vi "NIMS_DF_iir_grpdelay.vi"(5 "r":dbl=0.9999, 6 "w":dbl[](array[numeric]), 7 "grp":dbl[](array[numeric]), 9 "e":dbl[](array[numeric]), 10 "f":dbl[](array[numeric]), 11 "n":i32) -> (0 "error":i32, 1 "offset":dbl=0.9999, 2 "a":dbl[](array[numeric]), 3 "b":dbl[](array[numeric]))   [LabVIEW 2017, in "NI_DigFilter_MathScript.lvlib"]
uses:
  <vilib>/addons/Digital Filter Design/NI_DigFilter_MathScript.lvlib
  <vilib>/addons/Digital Filter Design/NI_DigFilterLicensed.lvlib
panel:
  in  "reserved4":dbl=nan
  in  "reserved3":dbl[](array[numeric])
  in  "reserved2":dbl=20.0
  in  "reserved1":i32[](array[numeric])=[2, 128]
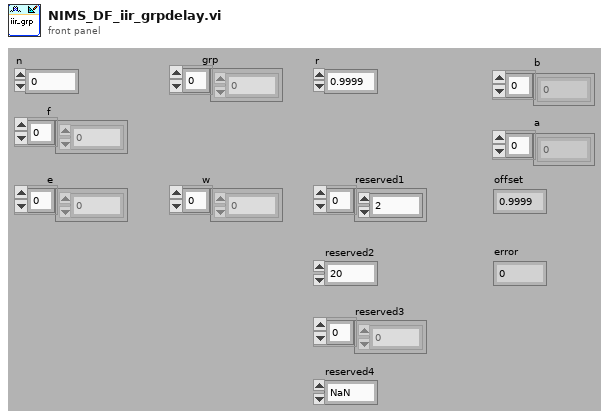
[diagram p1: front panel]
types:
  T1 = typedef "NI_DigFilterLicensed.lvlib/dfd_Group Delay_Band Spec.ctl" = cluster{"subband specs":cluster{"freq":dbl, "group delay":dbl, "weight":dbl}[]}
  T2 = typedef "NI_DigFilterLicensed.lvlib/DFD Filter Obj.ctl" = cluster{"mSRate_Fs":dbl, "mSRate_Version":string, "mSRate_Comments":string, "mSRate_OrgCoef":T3, "mSRate_CurCoef":T3, "mSRate_Quantized?":bool, "mSRate_QCoef":T3, "mSRate_QSettings":T5[], "mSRate_Order":i32, "mSRate_Scaling":cluster{"mSRate_ScaleByPowerOf2?":bool, "mSRate_ScaleType":T7}}
  T3 = typedef "NI_DigFilterLicensed.lvlib/DFD Filter Coef.ctl" = cluster{"type":T4, "gain":dbl, "coef a (k)":dbl[], "coef b (v)":dbl[]}
  T4 = typedef "NI_DigFilterLicensed.lvlib/DFD Filter Structure Type Selector.ctl" = enum16{"Undefined", "FIR Direct Form", "FIR Direct Form Transposed", "FIR Symmetric", "FIR Antisymmetric", "IIR Direct Form I", "IIR Direct Form I Transposed", "IIR Direct Form II", "IIR Direct Form II Transposed", "IIR Cascaded Second Order Sections Form I", "IIR Cascaded Second Order Sections Form I Transposed", "IIR Cascaded Second Order Sections Form II", "IIR Cascaded Second Order Sections Form II Transposed", "Lattice Allpass (basic sections)", "Lattice Allpass (one multiplier sections)", "Lattice Allpass (normalized sections)", "Lattice AR (basic sections)", "Lattice AR (one multiplier sections)", "Lattice AR (normalized sections)", "Lattice MA (minimum phase)", "Lattice MA (maximum phase)", "Lattice ARMA (basic sections)", "Lattice ARMA (one multiplier sections)", "Lattice ARMA (normalized sections)"}
  T5 = typedef "NI_DigFilterLicensed.lvlib/dfd_Internal Quantization Settings.ctl" = cluster{"source":T6, "wl":i16, "iwl":i16, "overflow mode":enum16{"Saturation", "Wrap"}, "rounding mode":enum16{"Nearest", "Truncation"}, "signed?":bool}
  T6 = typedef "NI_DigFilterLicensed.lvlib/dfd_Internal Quantization Srcs.ctl" = u16
  T7 = typedef "NI_DigFilterLicensed.lvlib/DFD Coef Norm Type.ctl" = enum16{"No Norm", "Time Domain 1-Norm", "Time Domain 2-Norm", "Time Domain Inf-Norm"}
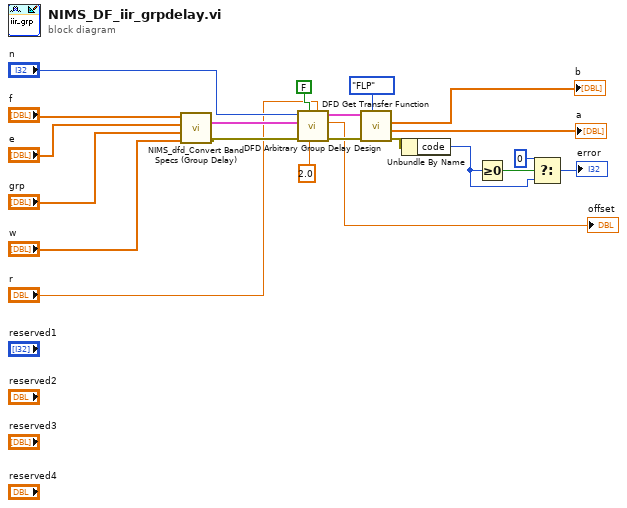
[diagram p0: block diagram]
diagram:
  n1 = call <vilib>:"NIMS_dfd_Convert Band Specs (Group Delay).vi"("W"="w", "Group Delay"="grp", "Edges"="e", "F"="f") -> ("error out"=w11:errorcluster, "band specs"=w12:T1[])  [unwired: 6 out]
  n2 = call <vilib>:"DFD Arbitrary Group Delay Design.vi"("pole radius constraint"="r", "fs [Hz]"=2.0, "integer offset? (T)"=FALSE, "error in (no error)"=w11, "band specs"=w12, "order"="n") -> ("error out"=w14:errorcluster, "offset"=→"offset":dbl, "filter out"=w15:T2)  [unwired: 3 out]
  n3 = call <vilib>:"DFD Get Transfer Function.vi"("type (FLP)"=enum16{"FLP", "FXP"}."FLP", "error in (no error)"=w14, "filter in"=w15) -> ("error out"=w5:errorcluster, "denominator"=→"a":dbl[], "numerator"=→"b":dbl[])  [unwired: 6 out]
  n4 = Unbundle By Name(w5) -> ("code"=w1:i32)
  n5 = Greater Or Equal To 0?(x=w1) -> (x >= 0?=w4:bool)
  n6 = Select(t=0 ("error"), s=w4, f=w1) -> (s? t:f=→"error":i32)
